vi "Prompt User for DSF Config File.vi"(8 "error in (no error)":errorcluster, 11 "Application Data in":T1) -> (0 "error out":errorcluster, 3 "Application Data out":T1)   [LabVIEW 2017, in "DSF Mini Explorer.lvlib"]
uses:
  DSF Mini Explorer.lvlib
  Application Data.ctl
  VeriStand/Data Sharing Custom Device/Source/DSF Core.lvlibp/Classes/Configuration/Configuration Session.lvclass
  View Mode.ctl
panel:
  # "App\nData"
  # "App\nData"
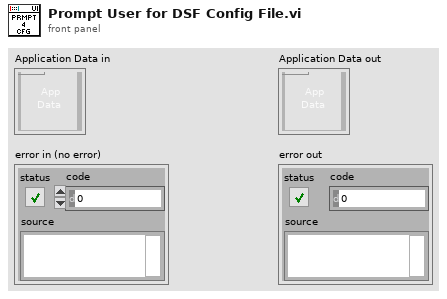
[diagram p1: front panel]
types:
  T1 = typedef "DSF Mini Explorer.lvlib/Application Data.ctl" = cluster{"Item Tree Control":refnum<vi>, "Value Tree Control":refnum<vi>, "DSF Refnum":refnum<class "Configuration Session.lvclass">, "Top-Level VI":refnum<vi>, "View State":T2, "menu reference":refnum<k9>}
  T2 = typedef "DSF Mini Explorer.lvlib/View Mode.ctl" = enum16{"Tree", "List"}
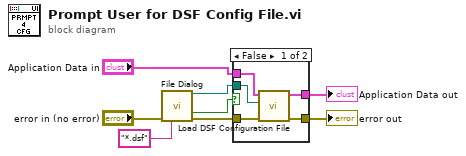
[diagram p0: block diagram]
diagram:
  n1 = call "File Dialog"("error in"="error in (no error)", "pattern (all files)"="*.dsf") -> ("selected path"=w2:path, "cancelled"=w3:bool, "error out"=w5:errorcluster)  [unwired: 10 in, 1 out]
  n2 = case shown="False" w3 {
    tunnel: w2 -> [w9 _]
    tunnel: [w11 w14] -> w6
    tunnel: w5 -> [w13 w15]
    tunnel: [w12 w15] -> w7
    tunnel: "Application Data in" -> [w10 w14]
    frame False {
      n3 = call "Load DSF Configuration File.vi"("error in (no error)"=w13, "Path"=w9, "Application Refs"=w10) -> ("error out"=w12:errorcluster, "Application Data out"=w11:T1)  [unwired: 7 in]
    }
    frame True {
    }
  }
  "error out" <- w7
  "Application Data out" <- w6
